vi "二维数组排序(U8).vi"(1 "数组输入":u8[][](array[numeric])) -> (0 "数组输出":u8[][](array[numeric]))   [LabVIEW 2014, in "数组操作.lvlib"]
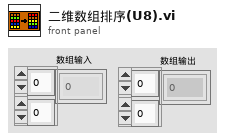
[diagram p1: front panel]
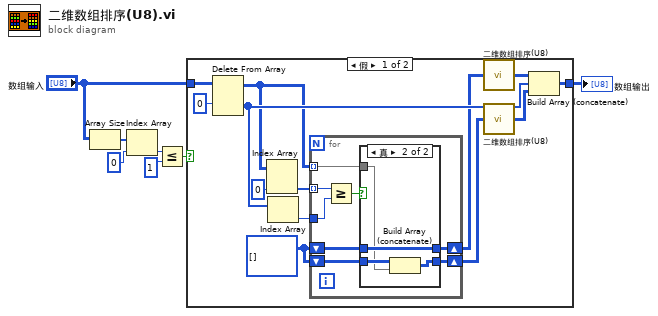
[diagram p0: block diagram]
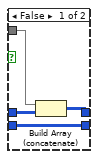
[diagram p2: hidden frame]
diagram:
  n1 = Array Size(array="数组输入") -> (size(s)=w3:i32[])
  n2 = Index Array(array=w3, index=0 ("y")) -> (element=w4:i32)
  n3 = Less Or Equal?(x=w4, y=1) -> (x <= y?=w7:bool)
  n4 = case shown="假" w7 {
    tunnel: "数组输入" -> [w19 w37]
    tunnel: [w12 w37] -> w5
    frame False {
      w17 = u8[][] [] ("数组")
      n5 = Delete From Array(array=w19, index (row)=0 ("索引")) -> (deleted portion=w20:u8[], array with subset deleted=w9:u8[][])  [unwired: 2 in]
      n6 = Index Array(array=w9, index (col)=0 ("禁用的索引 (列)")) -> (element=w11:u8[])  [unwired: 1 in]
      n7 = Index Array(array=w20) -> (element=w8:u8)  [unwired: 1 in]
      n8 = for {
        shift-right: [w25] -> w14
        shift-left: w17 -> [w24]
        shift-right: [w26] -> w13
        shift-left: w17 -> [w27]
        tunnel: w11 -> [w23] mode=indexing
        tunnel: w9 -> [w22] mode=indexing
        tunnel: w8 -> [w21]
        n9 = Greater Or Equal?(x=w23, y=w21) -> (x >= y?=w28:bool)
        n10 = case shown="真" w28 {
          tunnel: w27 -> [w30 w36]
          tunnel: [w30 w35] -> w26
          tunnel: [w32 w34] -> w25
          tunnel: w24 -> [w31 w34]
          tunnel: w22 -> [w29 w33]
          frame False {
            n11 = Build Array (concatenate)(w29, w31) -> (w32:u8[][])
          }
          frame True {
            n12 = Build Array (concatenate)(w36, w33) -> (w35:u8[][])
          }
        }
      }
      n13 = call "二维数组排序(U8).vi"("数组输入"=w14) -> ("数组输出"=w16:u8[][])
      n14 = call "二维数组排序(U8).vi"("数组输入"=w13) -> ("数组输出"=w15:u8[][])
      n15 = Build Array (concatenate)(w16, w20, w15) -> (w12:u8[][])
    }
    frame True {
    }
  }
  "数组输出" <- w5
